vi "VdDigitalControl_Create.vi"(8 "Error In":errorcluster, 11 "reference in":refnum<class "VdDigitalControl.lvclass">) -> (0 "Error Out":errorcluster, 3 "reference out":refnum<class "VdDigitalControl.lvclass">)   [LabVIEW 2020, in "VdDigitalControl.lvclass"]
uses:
  VdDigitalControl.lvclass
  VdDigitalControl.lvclass/VdDigitalControl.ctl
  VdInstrument_class/VdInstrument.lvclass
  C:/Projects/OpenGDS_DesignPatterns/Factory1/VdInstrument_class/VdInstrument.lvclass
  C:/Projects/OpenGDS_DesignPatterns/Factory1/VdDigitalControl_class/VdDigitalControl.lvclass
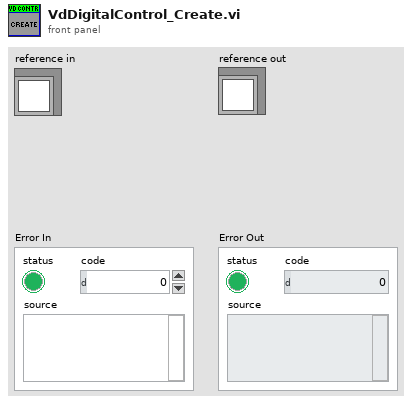
[diagram p1: front panel]
types:
  T1 = typedef "VdDigitalControl.lvclass/ObjectAttributes.ctl" = cluster{"CurrentState":bool}
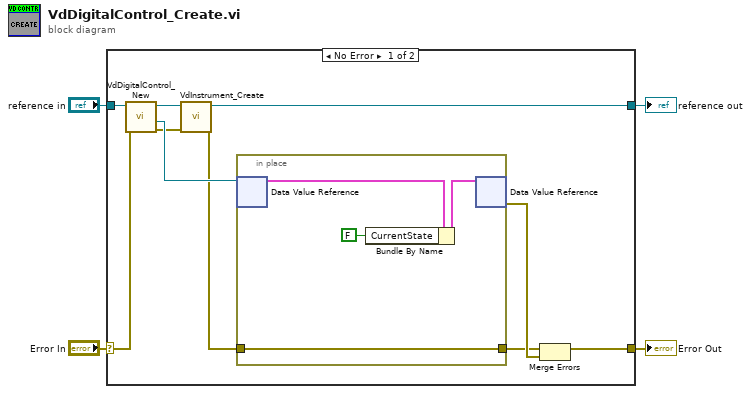
[diagram p0: block diagram]
diagram:
  n1 = case shown="No Error" "Error In" {
    selector: "Error In" -> [w10 w20]
    tunnel: [w8 w20] -> w3
    tunnel: "reference in" -> [w12 w19]
    tunnel: [w7 w19] -> w1
    frame No Error {
      n2 = call "VdDigitalControl_New.vi"("error in (no error)"=w10, "reference in"=w12) -> ("error out"=w11:errorcluster, "DVRRefOut"=w14:refnum<data-value>, "reference out"=w13:refnum<class "VdDigitalControl.lvclass">)  [unwired: 6 in, 1 out]
      n3 = call "VdInstrument_Create.vi"("Error In"=w11, "reference in"=w13) -> ("Error Out"=w6:errorcluster, "reference out"=w7:refnum<class "VdDigitalControl.lvclass">)  [unwired: 8 in]
      n4 = in-place {
        in-place-border: w6 -> [w15]
        in-place-border: [w15] -> w5
        n5 = in-place-dvr #1(w14) -> (w17:T1)  [unwired: 1 out]
        n6 = Bundle By Name(cluster=w17, "CurrentState"=FALSE) -> (w18:T1)
        n7 = in-place-dvr #1(w18) -> (w9:errorcluster)  [unwired: 1 out]
      }
      n8 = Merge Errors(w5, w9) -> (w8:errorcluster)
    }
    frame Error {
    }
  }
  "Error Out" <- w3
  "reference out" <- w1
